vi "Copy Packaging Components.vi"(0 "Primary destination path":path, 5 "Template Path":path, 11 "error in (no error)":errorcluster) -> (4 "Package Files":path[](array[path]), 15 "error out":errorcluster)   [LabVIEW 2021, in "Packager Helpers.lvlib"]
uses:
  Packager Helpers.lvlib
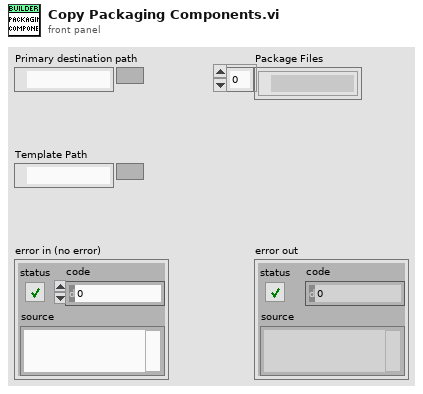
[diagram p1: front panel]
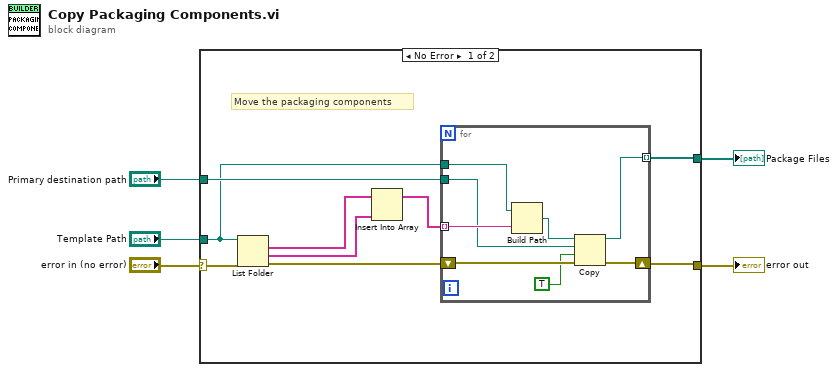
[diagram p0: block diagram]
diagram:
  n1 = case shown="No Error" "error in (no error)" {
    selector: "error in (no error)" -> [w8 w23]
    tunnel: "Template Path" -> [w6 _]
    tunnel: [w9 w23] -> w3
    tunnel: [w10 _] -> w2
    tunnel: "Primary destination path" -> [w7 _]
    frame No Error {
      # "Move the packaging components"
      n2 = List Folder(path=w6, error in=w8) -> (filenames=w11:string[], folder names=w12:string[], error out=w14:errorcluster)  [unwired: 2 in, 1 out]
      n3 = Insert Into Array(array=w11, new element=w12) -> (w13:string[])  [unwired: 1 in]
      n4 = for {
        shift-right: [w21] -> w9
        shift-left: w14 -> [w22]
        tunnel: w13 -> [w20] mode=indexing
        tunnel: [w18] -> w10 mode=indexing
        tunnel: w7 -> [w16]
        tunnel: w6 -> [w15]
        n5 = Build Path(base path=w15, name or relative path=w20) -> (appended path=w19:path)
        n6 = Copy(8:w22, 9:TRUE ("overwrite (F)"), 10:w16, 11:w19) -> (0:w21:errorcluster, 3:w18:path)  [unwired: 1 in, 1 out]
      }
    }
    frame Error {
    }
  }
  "error out" <- w3
  "Package Files" <- w2
